vi "Home Top Level.vi"   [LabVIEW 2020, in "Endigit.lvlib"]
doc: "Places the origin of the front panel of the top level VI at the top left of the panel.\n\nAuthored by Robert C. Mortensen\nrobert@endigit.com\n\nCopyright (c) 2015, Endigit, Inc."
uses:
  Endigit.lvlib
  <vilib>/Utility/miscctls.llb/LVPointTypeDef.ctl
types:
  T1 = typedef "LVPointTypeDef.ctl" = cluster{"Horizontal":i16, "Vertical":i16}
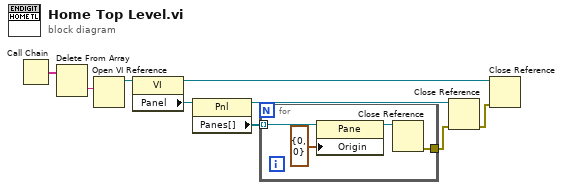
[diagram p0: block diagram]
diagram:
  n1 = Call Chain() -> (call chain=w7:string[])
  n2 = Delete From Array(array=w7) -> (deleted portion=w6:string)  [unwired: 2 in, 1 out]
  n3 = Open VI Reference(vi path=w6) -> (vi reference=w5:refnum<vi>)  [unwired: 5 in, 1 out]
  n4 = property class="VI"(reference=w5) -> (reference out=w3:refnum<vi>, "Panel"=w9:refnum<vi>)  [unwired: 1 in, 1 out]
  n5 = property class="Pnl"(reference=w9) -> (reference out=w4:refnum<vi>, "Panes[]"=w8:refnum<vi>[])  [unwired: 1 in, 1 out]
  n6 = for {
    tunnel: w8 -> [w13] mode=indexing
    tunnel: [w10] -> w1
    n7 = property class="Pane"(reference=w13, "Origin"=T1 {"Horizontal"=0, "Vertical"=0} ("Horizontal Scrollbar Visibility")) -> (reference out=w11:refnum<vi>)  [unwired: 1 in, 1 out]
    n8 = Close Reference(reference=w11) -> (error out=w10:errorcluster)  [unwired: 1 in]
  }
  n9 = Close Reference(reference=w4, error in (no error)=w1) -> (error out=w2:errorcluster)
  n10 = Close Reference(reference=w3, error in (no error)=w2) -> ()  [unwired: 1 out]
